vi "Outcome - When Set Explicitly - Returns Configured Value.vi"() -> ()   [LabVIEW 2017, in "Test Result.Tests.lvlib"]
uses:
  Test Result.Tests.lvlib
  Test Result/Test Result.lvclass
  Test Outcome.ctl
  Test Result/Test Result.lvclass/Test Result.ctl
  Test Result/Set Outcome.vi
  Test Result/Get Outcome.vi
  <vilib>/PNR/Transparent Assertions/Transparent Assertions/Transparent Assertions.lvlib
panel:
  out "error out":errorcluster
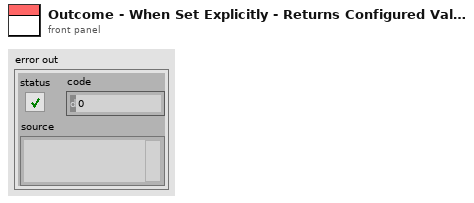
[diagram p1: front panel]
types:
  T1 = typedef "Test Outcome.ctl" = enum16{"None", "Passed", "Failed"}
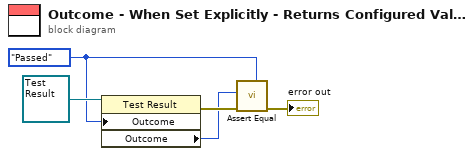
[diagram p0: block diagram]
diagram:
  w2 = Test_Outcome."Passed" ("Test Outcome")
  n1 = property class="Test Result"(reference=refnum<class "Test Result.lvclass"> refnum ("Test Result"), "Outcome"=w2) -> (error out=w4:errorcluster, "Outcome"=w1:T1)  [unwired: 1 in, 1 out]
  n2 = call <vilib>:"Assert Equal.vi"("Expected"=w2, "error in (no error)"=w4, "Actual"=w1) -> ("error out"=→"error out":errorcluster)  [unwired: 8 in]
